vi "ArrowUpDown.vi"(5 "Remove Layer":refnum<vi>, 7 "# Layers":i32, 8 "error in (no error)":errorcluster, 9 "Arrow Down":refnum<vi>, 10 "Arrow Up":refnum<vi>, 11 "FakedArray in":refnum<class "FakedArray.lvclass">) -> (0 "error out":errorcluster, 3 "FakedArray out":refnum<class "FakedArray.lvclass">)   [LabVIEW 2021, in "FakedArray.lvclass"]
uses:
  <resource>/plugins/NIIconEditor/Class/FakedArray/FakedArray.lvclass
  <resource>/plugins/NIIconEditor/Controls/Arrow Down.ctl
  <resource>/plugins/NIIconEditor/Class/FakedArray/FakedArray.lvclass/FakedArray.ctl
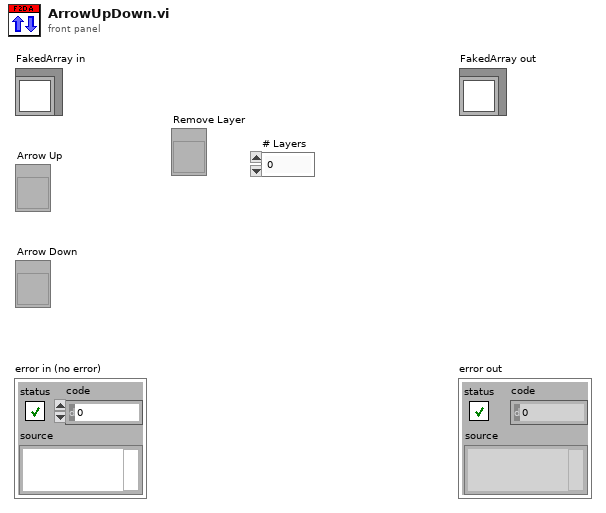
[diagram p1: front panel]
types:
  T1 = typedef "ToMoreSpecific_Faked2DArray.ctl" = enum16{"Framework Templates", "Layer List"}
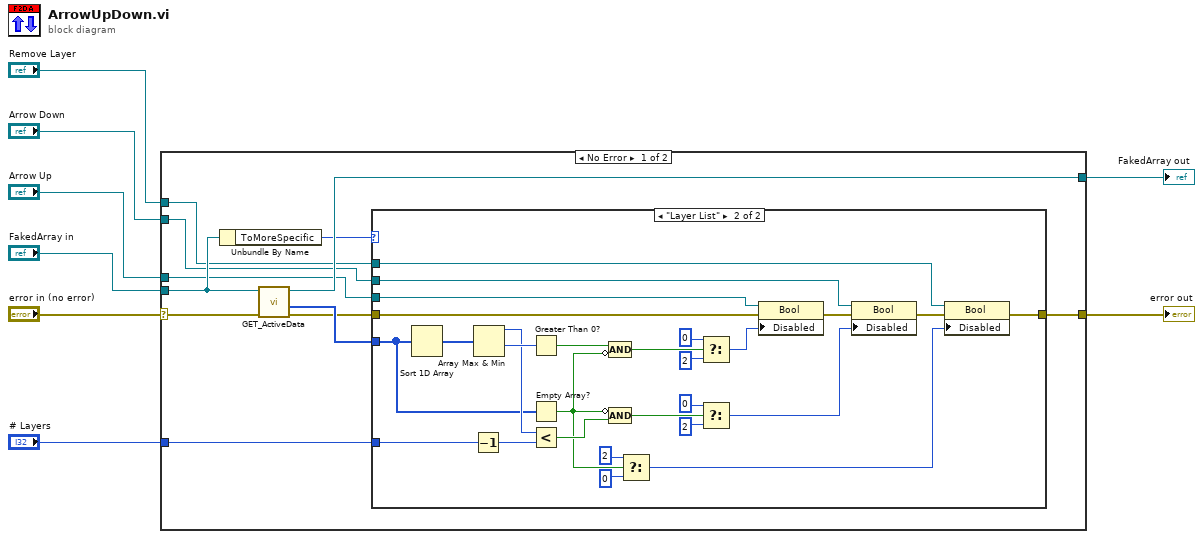
[diagram p0: block diagram]
diagram:
  n1 = case shown="No Error" "error in (no error)" {
    selector: "error in (no error)" -> [w14 w49]
    tunnel: [w18 w49] -> w7
    tunnel: [w17 w48] -> w5
    tunnel: "FakedArray in" -> [w15 w48]
    tunnel: "# Layers" -> [w19 _]
    tunnel: "Arrow Up" -> [w11 _]
    tunnel: "Arrow Down" -> [w10 _]
    tunnel: "Remove Layer" -> [w9 _]
    frame No Error {
      n2 = Unbundle By Name(w15) -> ("ToMoreSpecific"=w12:T1)
      n3 = call-dynamic "GET_ActiveData.vi"("error in (no error)"=w14, "FakedArray in"=w15) -> ("error out"=w13:errorcluster, "Active Data []"=w16:i32[], "FakedArray out"=w17:refnum<class "FakedArray.lvclass">)  [unwired: 7 out]
      n4 = case shown="\"Layer List\"" w12 {
        tunnel: w13 -> [w20 w32]
        tunnel: w11 -> [_ w45]
        tunnel: w10 -> [_ w41]
        tunnel: w19 -> [_ w25]
        tunnel: [w20 w28] -> w18
        tunnel: w16 -> [_ w31]
        tunnel: w9 -> [_ w30]
        frame "Framework Templates", Default {
        }
        frame "Layer List" {
          n5 = Sort 1D Array(array=w31) -> (sorted array=w47:i32[])
          n6 = Decrement(x=w25) -> (x-1=w37:i32)
          n7 = Array Max & Min(array=w47) -> (max value=w36:i32, min value=w46:i32)  [unwired: 2 out]
          n8 = Greater Than 0?(x=w46) -> (x > 0?=w34:bool)
          n9 = Empty Array?(array=w31) -> (empty?=w22:bool)
          n10 = Less?(x=w36, y=w37) -> (x < y?=w33:bool)
          n11 = Compound Arithmetic op=AND(w34, invert w22) -> (w27:bool)
          n12 = Compound Arithmetic op=AND(invert w22, w33) -> (w26:bool)
          n13 = Select(t=u8 2 ("Disabled"), s=w22, f=u8 0 ("Disabled")) -> (s? t:f=w21:u8)
          n14 = Select(t=u8 0 ("Disabled"), s=w27, f=u8 2 ("Disabled")) -> (s? t:f=w42:u8)
          n15 = Select(t=u8 0 ("Disabled"), s=w26, f=u8 2 ("Disabled")) -> (s? t:f=w35:u8)
          n16 = property class="Bool"(reference=w45, error in=w32, "Disabled"=w42) -> (error out=w40:errorcluster)  [unwired: 1 out]
          n17 = property class="Bool"(reference=w41, error in=w40, "Disabled"=w35) -> (error out=w29:errorcluster)  [unwired: 1 out]
          n18 = property class="Bool"(reference=w30, error in=w29, "Disabled"=w21) -> (error out=w28:errorcluster)  [unwired: 1 out]
        }
      }
    }
    frame Error {
    }
  }
  "error out" <- w7
  "FakedArray out" <- w5
